vi "main_重写.vi"() -> ()   [LabVIEW 2022 SP3]
uses:
  <vilib>/Instr/_visa.llb/VISA Configure Serial Port (Instr).vi
panel:
  in  "ki2":dbl
  in  "ki1":dbl=0.15
  in  "kp1":dbl=75.0
  in  "kp2":dbl=30.0
  in  "kd2":dbl=2000.0
  in  "kd1":dbl=260.0
  in  "匀速转动":bool
  in  "自动起摆":bool
  in  "自平衡":bool
  out "ENC":dbl
  out "ADC":dbl
  out "ENC":u16(graph)
  out "ADC":u16(graph)
  in  "端口":refnum<visa-resource-name> caption="VISA资源名称"
  # "串口配置"
  # "仪表盘"
  # "控制台"
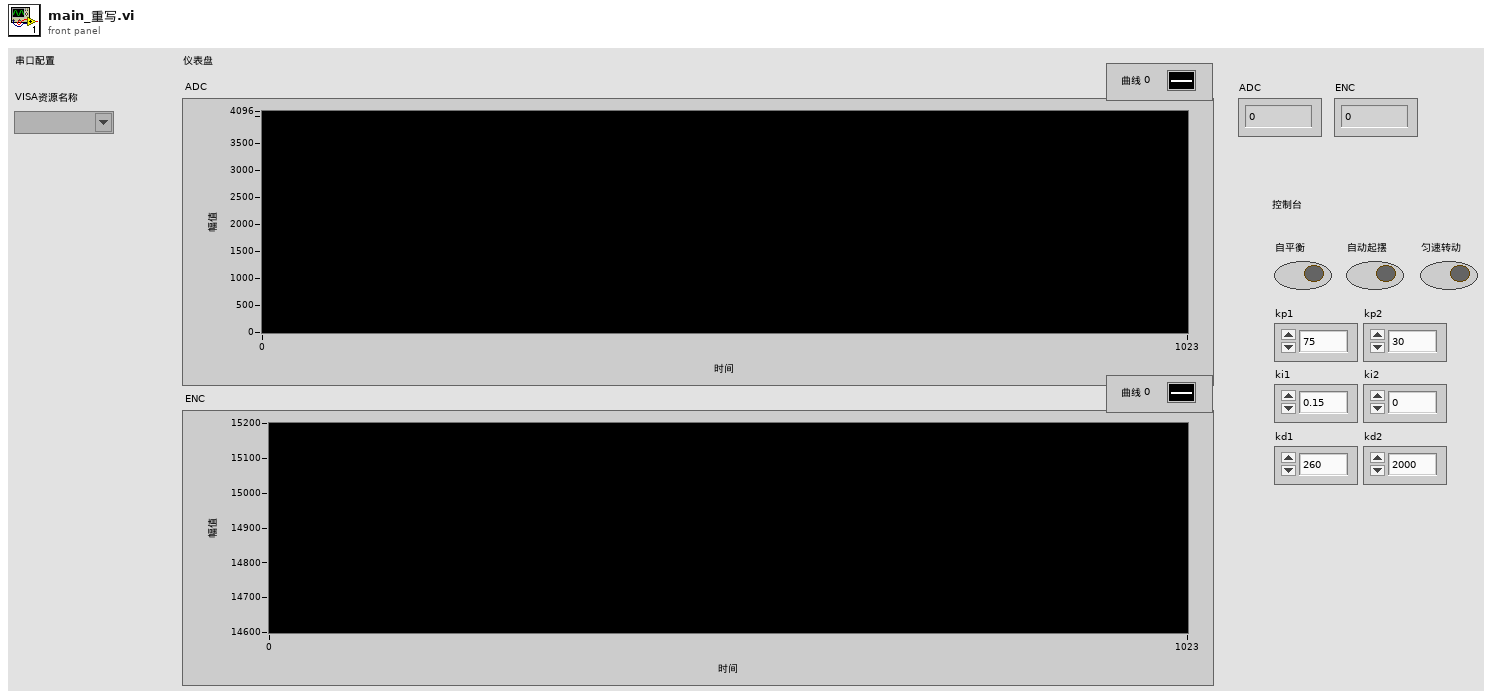
[diagram p1: front panel]
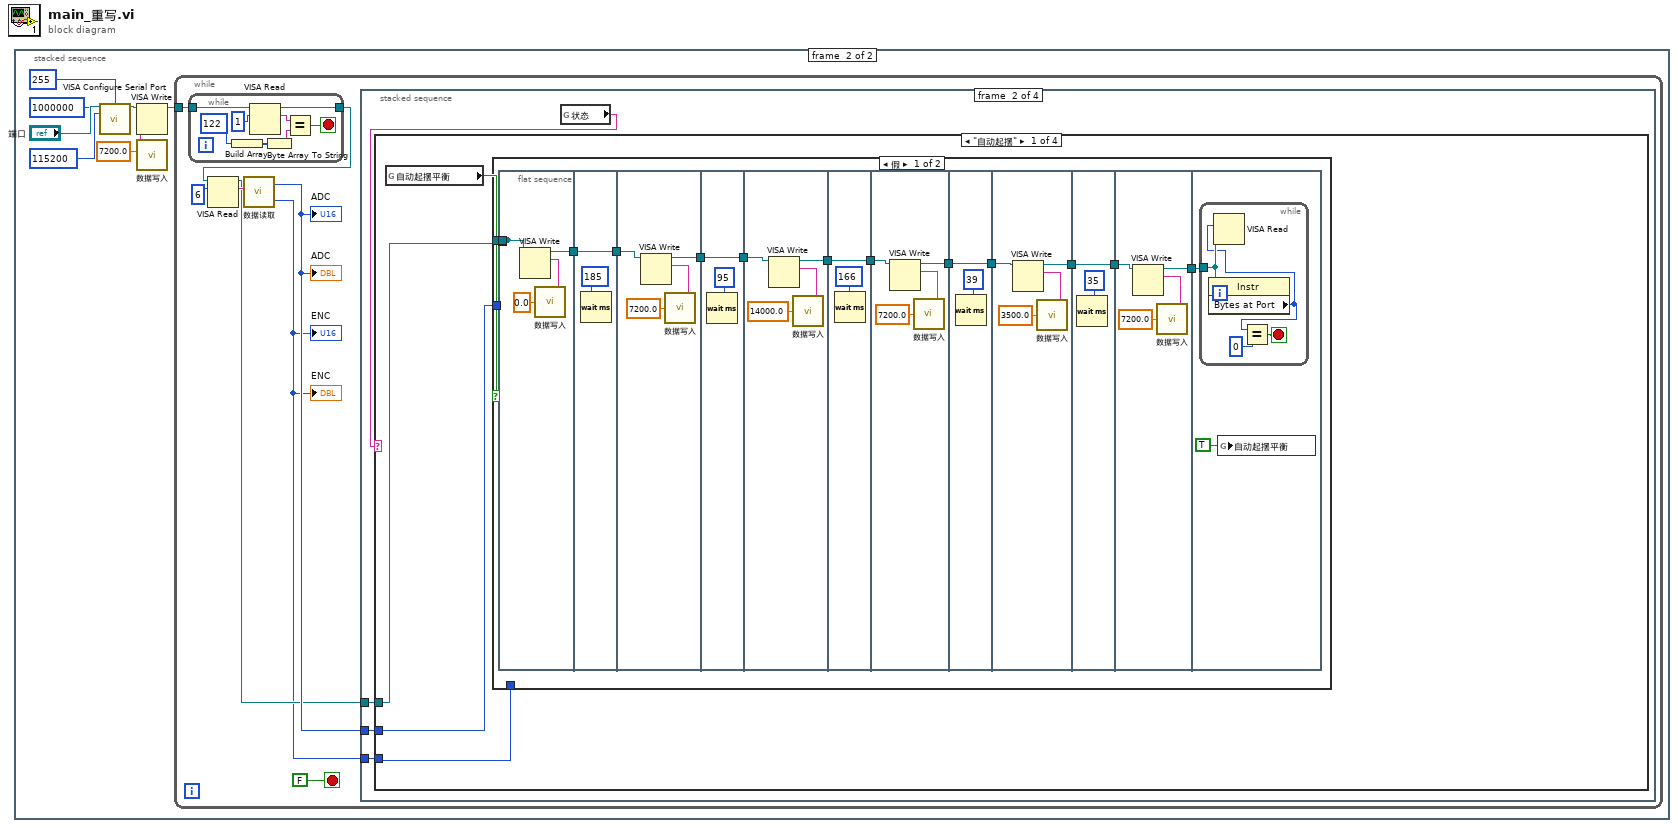
[diagram p0: block diagram]
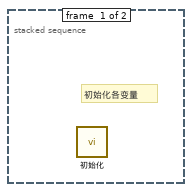
[diagram p2: hidden frame]
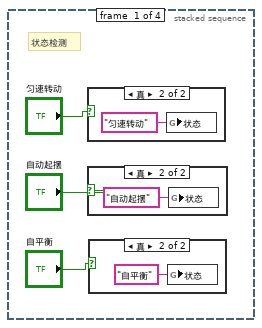
[diagram p3: hidden frame]
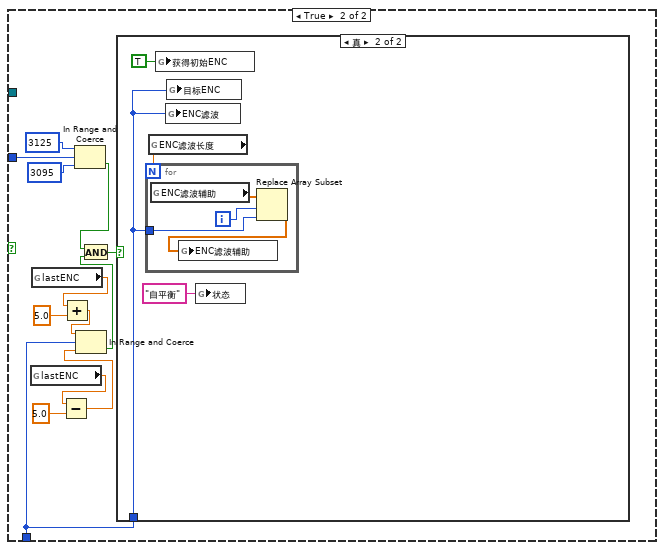
[diagram p7: hidden frame]
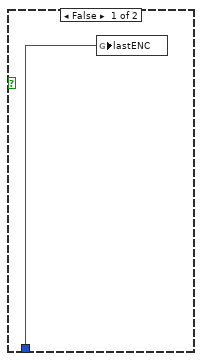
[diagram p8: hidden frame]
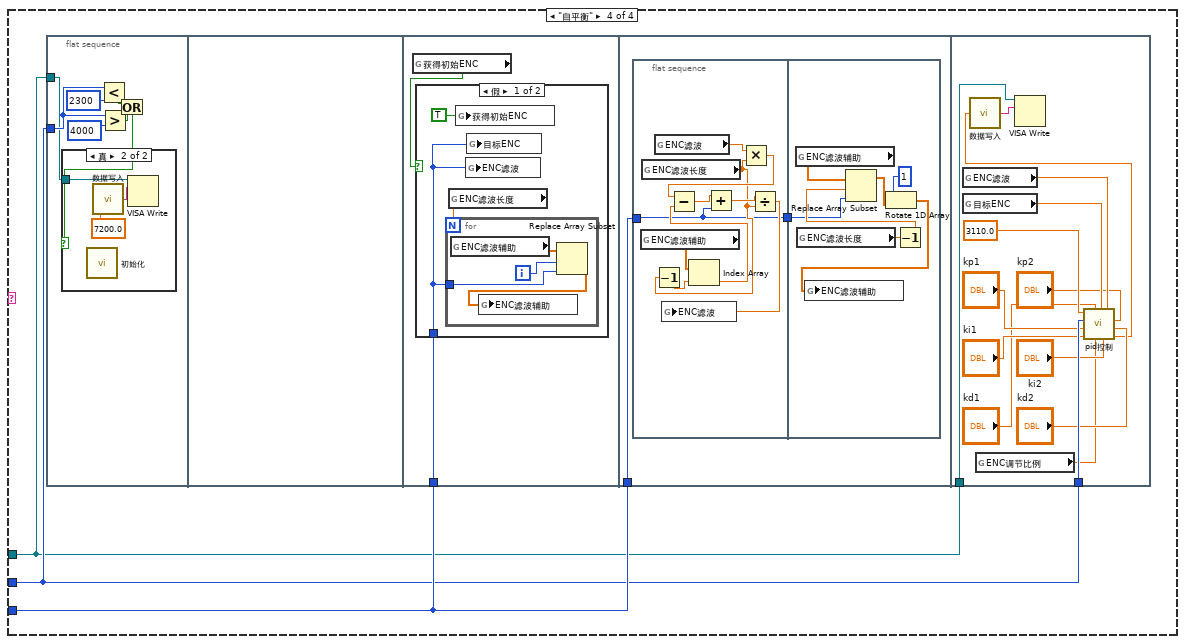
[diagram p11: hidden frame]
diagram:
  n1 = stacked-sequence {
    frame #0 {
      # "初始化各变量"
      n2 = call "初始化.vi"() -> ()  [unwired: 12 in]
    }
    frame #1 {
      n3 = call-poly "VISA Configure Serial Port"("VISA resource name"="端口", "timeout (10sec)"=u32 1000000, "termination char\n(0xA = '\\n' = LF)"=u8 255 ("termination char\n(0xA = '\\n' = LF)"), "baud rate (9600)"=u32 115200) -> ("VISA resource name out"=w2:refnum<visa-resource-name>)  [unwired: 10 in, 1 out]
      n4 = call "数据写入.vi"("PWM"=7200.0) -> ("输出"=w4:string)
      n5 = VISA Write(VISA resource name=w2, write buffer=w4) -> (VISA resource name out=w1:refnum<visa-resource-name>)  [unwired: 1 in, 2 out]
      n6 = while {
        tunnel: w1 -> [w16]
        stop <- FALSE stop-if-true
        n7 = while {
          tunnel: w16 -> [w167]
          tunnel: [w161] -> w15
          stop <- w162 stop-if-true
          n8 = Build Array(u8 122) -> (w164:u8[])
          n9 = VISA Read(VISA resource name=w167, byte count=u32 1 ("字节总数")) -> (VISA resource name out=w161:refnum<visa-resource-name>, read buffer=w160:string)  [unwired: 1 in, 2 out]
          n10 = Byte Array To String(unsigned byte array=w164) -> (string=w163:string)
          n11 = Equal?(x=w160, y=w163) -> (x = y?=w162:bool)
        }
        n12 = VISA Read(VISA resource name=w15, byte count=u32 6 ("字节总数")) -> (VISA resource name out=w11:refnum<visa-resource-name>, read buffer=w13:string)  [unwired: 1 in, 2 out]
        n13 = call "数据读取.vi"("字符串"=w13) -> ("ADC"=w12:u16, "ENC"=w10:u16)
        "ADC" <- w12
        "ADC" <- w12
        "ENC" <- w10
        "ENC" <- w10
        n14 = stacked-sequence {
          tunnel: w12 -> [_ w25 _ _]
          tunnel: w11 -> [_ w24 _ _]
          tunnel: w10 -> [_ w23 _ _]
          frame #0 {
            # "状态检测"
            n15 = case shown="真" "匀速转动" {
              frame False {
              }
              frame True {
                n16 = global write "全局变量.vi" "状态"("匀速转动" ("状态")) -> ()
              }
            }
            n17 = case shown="真" "自动起摆" {
              frame False {
              }
              frame True {
                n18 = global write "全局变量.vi" "状态"("自动起摆" ("状态")) -> ()
              }
            }
            n19 = case shown="真" "自平衡" {
              frame False {
              }
              frame True {
                n20 = global write "全局变量.vi" "状态"("自平衡" ("状态")) -> ()
              }
            }
          }
          frame #1 {
            n21 = global read "全局变量.vi" "状态"() -> (w26:string)
            n22 = case shown="\"自动起摆\"" w26 {
              tunnel: w25 -> [w28 _ _ w106]
              tunnel: w24 -> [w29 _ _ w105]
              tunnel: w23 -> [w27 _ _ w107]
              frame "自动起摆" {
                n23 = global read "全局变量.vi" "自动起摆平衡"() -> (w30:bool)
                n24 = case shown="假" w30 {
                  tunnel: w29 -> [w31 _]
                  tunnel: w28 -> [_ w95]
                  tunnel: w27 -> [_ w90]
                  frame False {
                    n25 = flat-sequence {
                      tunnel: [w43] -> _
                      tunnel: [w44] -> w42
                      tunnel: w31 -> [w43]
                      tunnel: [w47] -> w41
                      tunnel: w42 -> [w47]
                      tunnel: w41 -> [w50]
                      tunnel: [w49] -> w40
                      tunnel: [w53] -> w39
                      tunnel: w40 -> [w53]
                      tunnel: w39 -> [w56]
                      tunnel: [w55] -> w38
                      tunnel: [w59] -> w37
                      tunnel: w38 -> [w59]
                      tunnel: w37 -> [w62]
                      tunnel: [w61] -> w36
                      tunnel: [w65] -> w35
                      tunnel: w36 -> [w65]
                      tunnel: w35 -> [w68]
                      tunnel: [w67] -> w34
                      tunnel: [w71] -> w33
                      tunnel: w34 -> [w71]
                      tunnel: w33 -> [w74]
                      tunnel: [w73] -> w32
                      tunnel: w32 -> [w78]
                      frame #0 {
                        n26 = call "数据写入.vi"("PWM"=0.0) -> ("输出"=w45:string)
                        n27 = VISA Write(VISA resource name=w43, write buffer=w45) -> (VISA resource name out=w44:refnum<visa-resource-name>)  [unwired: 1 in, 2 out]
                      }
                      frame #1 {
                        n28 = Wait (ms)(milliseconds to wait=u32 185 ("等待时间（毫秒）")) -> ()  [unwired: 1 out]
                      }
                      frame #2 {
                        n29 = call "数据写入.vi"("PWM"=7200.0) -> ("输出"=w51:string)
                        n30 = VISA Write(VISA resource name=w50, write buffer=w51) -> (VISA resource name out=w49:refnum<visa-resource-name>)  [unwired: 1 in, 2 out]
                      }
                      frame #3 {
                        n31 = Wait (ms)(milliseconds to wait=u32 95 ("等待时间（毫秒）")) -> ()  [unwired: 1 out]
                      }
                      frame #4 {
                        n32 = call "数据写入.vi"("PWM"=14000.0) -> ("输出"=w57:string)
                        n33 = VISA Write(VISA resource name=w56, write buffer=w57) -> (VISA resource name out=w55:refnum<visa-resource-name>)  [unwired: 1 in, 2 out]
                      }
                      frame #5 {
                        n34 = Wait (ms)(milliseconds to wait=u32 166 ("等待时间（毫秒）")) -> ()  [unwired: 1 out]
                      }
                      frame #6 {
                        n35 = call "数据写入.vi"("PWM"=7200.0) -> ("输出"=w63:string)
                        n36 = VISA Write(VISA resource name=w62, write buffer=w63) -> (VISA resource name out=w61:refnum<visa-resource-name>)  [unwired: 1 in, 2 out]
                      }
                      frame #7 {
                        n37 = Wait (ms)(milliseconds to wait=u32 39 ("等待时间（毫秒）")) -> ()  [unwired: 1 out]
                      }
                      frame #8 {
                        n38 = call "数据写入.vi"("PWM"=3500.0) -> ("输出"=w69:string)
                        n39 = VISA Write(VISA resource name=w68, write buffer=w69) -> (VISA resource name out=w67:refnum<visa-resource-name>)  [unwired: 1 in, 2 out]
                      }
                      frame #9 {
                        n40 = Wait (ms)(milliseconds to wait=u32 35 ("等待时间（毫秒）")) -> ()  [unwired: 1 out]
                      }
                      frame #10 {
                        n41 = call "数据写入.vi"("PWM"=7200.0) -> ("输出"=w75:string)
                        n42 = VISA Write(VISA resource name=w74, write buffer=w75) -> (VISA resource name out=w73:refnum<visa-resource-name>)  [unwired: 1 in, 2 out]
                      }
                      frame #11 {
                        n43 = while {
                          tunnel: w78 -> [w82]
                          stop <- w81 stop-if-true
                          n44 = property class="Instr"(reference=w82) -> ("Bytes at Port"=w80:u32)  [unwired: 1 in, 2 out]
                          n45 = VISA Read(VISA resource name=w82, byte count=w80) -> ()  [unwired: 1 in, 4 out]
                          n46 = Equal?(x=w80, y=u32 0) -> (x = y?=w81:bool)
                        }
                        n47 = global write "全局变量.vi" "自动起摆平衡"(TRUE ("自动起摆平衡")) -> ()
                      }
                    }
                  }
                  frame True {
                    n48 = global read "全局变量.vi" "lastENC"() -> (w86:dbl)
                    n49 = global read "全局变量.vi" "lastENC"() -> (w89:dbl)
                    n50 = Subtract(x=w86, y=5.0) -> (x-y=w85:dbl)
                    n51 = Add(x=w89, y=5.0) -> (x+y=w84:dbl)
                    n52 = In Range and Coerce(upper limit=u16 3125 ("上限"), x=w95, lower limit=u16 3095 ("下限")) -> (In Range?=w91:bool)  [unwired: 1 out]
                    n53 = In Range and Coerce(upper limit=w84, x=w90, lower limit=w85) -> (In Range?=w83:bool)  [unwired: 1 out]
                    n54 = And(x=w91, y=w83) -> (x .and. y?=w92:bool)
                    n55 = case shown="真" w92 {
                      tunnel: w90 -> [w96 w98]
                      frame False {
                        n56 = global write "全局变量.vi" "lastENC"(w96) -> ()
                      }
                      frame True {
                        n57 = global read "全局变量.vi" "ENC滤波长度"() -> (w99:dbl)
                        n58 = for {
                          N: w99 -> [_]
                          tunnel: w98 -> [w101]
                          i -> [w103]
                          n59 = global read "全局变量.vi" "ENC滤波辅助"() -> (w104:dbl[])
                          n60 = Replace Array Subset(array=w104, new element=w101, index=w103) -> (w102:dbl[])
                          n61 = global write "全局变量.vi" "ENC滤波辅助"(w102) -> ()
                        }
                        n62 = global write "全局变量.vi" "获得初始ENC"(TRUE ("获得初始ENC")) -> ()
                        n63 = global write "全局变量.vi" "ENC滤波"(w98) -> ()
                        n64 = global write "全局变量.vi" "目标ENC"(w98) -> ()
                        n65 = global write "全局变量.vi" "状态"("自平衡" ("状态")) -> ()
                      }
                    }
                  }
                }
              }
              frame "匀速转动" {
              }
              frame "自由态", Default {
              }
              frame "自平衡" {
                n66 = flat-sequence {
                  tunnel: w106 -> [w110]
                  tunnel: w105 -> [w108]
                  tunnel: w107 -> [w118]
                  tunnel: w107 -> [w128]
                  tunnel: w106 -> [w158]
                  tunnel: w105 -> [w147]
                  frame #0 {
                    n67 = Less?(x=w110, y=u16 2300) -> (x < y?=w112:bool)
                    n68 = Greater?(x=w110, y=u16 4000) -> (0:w111:bool)
                    n69 = Or(x=w112, y=w111) -> (x .or. y?=w109:bool)
                    n70 = case shown="真" w109 {
                      tunnel: w108 -> [_ w117]
                      frame False {
                      }
                      frame True {
                        n71 = call "初始化.vi"() -> ()  [unwired: 12 in]
                        n72 = call "数据写入.vi"("PWM"=7200.0) -> ("输出"=w115:string)
                        n73 = VISA Write(VISA resource name=w117, write buffer=w115) -> ()  [unwired: 1 in, 3 out]
                      }
                    }
                  }
                  frame #1 {
                  }
                  frame #2 {
                    n74 = global read "全局变量.vi" "获得初始ENC"() -> (w119:bool)
                    n75 = case shown="假" w119 {
                      tunnel: w118 -> [w120 _]
                      frame False {
                        n76 = global read "全局变量.vi" "ENC滤波长度"() -> (w121:dbl)
                        n77 = for {
                          N: w121 -> [_]
                          tunnel: w120 -> [w123]
                          i -> [w125]
                          n78 = global read "全局变量.vi" "ENC滤波辅助"() -> (w126:dbl[])
                          n79 = Replace Array Subset(array=w126, new element=w123, index=w125) -> (w124:dbl[])
                          n80 = global write "全局变量.vi" "ENC滤波辅助"(w124) -> ()
                        }
                        n81 = global write "全局变量.vi" "获得初始ENC"(TRUE ("获得初始ENC")) -> ()
                        n82 = global write "全局变量.vi" "ENC滤波"(w120) -> ()
                        n83 = global write "全局变量.vi" "目标ENC"(w120) -> ()
                      }
                      frame True {
                      }
                    }
                  }
                  frame #3 {
                    n84 = flat-sequence {
                      tunnel: w128 -> [w129]
                      tunnel: [w129] -> w127
                      tunnel: w127 -> [w142]
                      frame #0 {
                        n85 = global read "全局变量.vi" "ENC滤波辅助"() -> (w137:dbl[])
                        n86 = global read "全局变量.vi" "ENC滤波长度"() -> (w131:dbl)
                        n87 = Decrement(x=w131) -> (x-1=w136:dbl)
                        n88 = global read "全局变量.vi" "ENC滤波"() -> (w138:dbl)
                        n89 = Index Array(array=w137, index=w136) -> (element=w134:dbl)
                        n90 = Multiply(x=w138, y=w131) -> (x*y=w135:dbl)
                        n91 = Subtract(x=w135, y=w134) -> (x-y=w133:dbl)
                        n92 = Add(x=w133, y=w129) -> (x+y=w132:dbl)
                        n93 = Divide(x=w132, y=w131) -> (x/y=w130:dbl)
                        n94 = global write "全局变量.vi" "ENC滤波"(w130) -> ()
                      }
                      frame #1 {
                        n95 = global read "全局变量.vi" "ENC滤波辅助"() -> (w145:dbl[])
                        n96 = global read "全局变量.vi" "ENC滤波长度"() -> (w144:dbl)
                        n97 = Decrement(x=w144) -> (x-1=w143:dbl)
                        n98 = Replace Array Subset(array=w145, new element=w142, index=w143) -> (w141:dbl[])
                        n99 = Rotate 1D Array(1:w141, 2:1 ("n")) -> (0:w139:dbl[])
                        n100 = global write "全局变量.vi" "ENC滤波辅助"(w139) -> ()
                      }
                    }
                  }
                  frame #4 {
                    n101 = global read "全局变量.vi" "ENC滤波"() -> (w153:dbl)
                    n102 = global read "全局变量.vi" "目标ENC"() -> (w154:dbl)
                    n103 = global read "全局变量.vi" "ENC调节比例"() -> (w146:dbl)
                    n104 = call "pid控制.vi"("kd2"="kd2", "kp2"="kp2", "当前ENC"=w153, "ki2"="ki2", "目标ENC"=w154, "ENC调节比例"=w146, "kd1"="kd1", "ki1"="ki1", "kp1"="kp1", "当前ADC"=w158, "目标ADC"=3110.0) -> ("PWM输出"=w149:dbl)
                    n105 = call "数据写入.vi"("PWM"=w149) -> ("输出"=w148:string)
                    n106 = VISA Write(VISA resource name=w147, write buffer=w148) -> ()  [unwired: 1 in, 3 out]
                  }
                }
              }
            }
          }
          frame #2 {
          }
          frame #3 {
          }
        }
      }
    }
  }
